vi "Sine.vi"() -> ()   [LabVIEW 2014]
panel:
  in  "Amount of points":dbl
  in  "Time between points":dbl(knob) scale=0.0..500.0
  in  "Points per cycle":dbl
  out "Waveform Chart":dbl(graph)
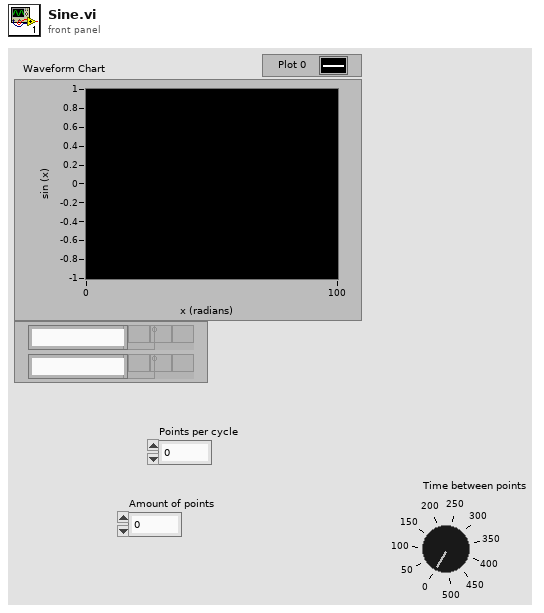
[diagram p1: front panel]
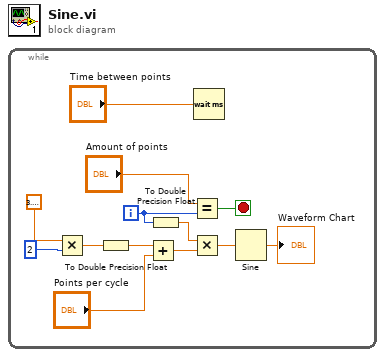
[diagram p0: block diagram]
diagram:
  n1 = while {
    i -> [w3]
    stop <- w2 stop-if-true
    n2 = Multiply(x=3.141592653589793, y=2) -> (x*y=w10:dbl)
    n3 = To Double Precision Float(number=w10) -> (double precision float=w9:dbl)
    n4 = Add(x=w9, y="Points per cycle") -> (x+y=w7:dbl)
    n5 = To Double Precision Float(number=w3) -> (double precision float=w6:dbl)
    n6 = Equal?(x="Amount of points", y=w3) -> (x = y?=w2:bool)
    n7 = Multiply(x=w6, y=w7) -> (x*y=w8:dbl)
    n8 = Wait (ms)(milliseconds to wait="Time between points") -> ()  [unwired: 1 out]
    n9 = Sine(x=w8) -> (sin(x)=→"Waveform Chart":dbl)
  }
